vi "PC Send Event.vi"(0 "PC Send Command":T1, 2 "Mode":T2, 7 "Flattened Data":string, 11 "Error In":errorcluster) -> (4 "PC Send Event":refnum<user-event>, 15 "Error Out":errorcluster)   [LabVIEW 2019]
uses:
  Event Mode.ctl
  PCsend RTrecv CMD.ctl
  PCsend RTrecv Cluster.ctl
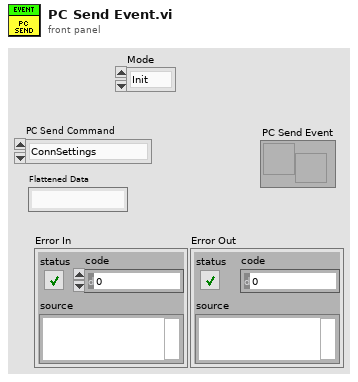
[diagram p1: front panel]
types:
  T1 = typedef "PCsend RTrecv CMD.ctl" = enum16{"ConnSettings", "Connect", "Stop", "Digital Outputs", "Analog Outputs", "Sweep Parameters", "Start Sweep", "Cal2RT", "Save Cal", "Load Cal"}
  T2 = typedef "Event Mode.ctl" = enum16{"Init", "Get", "Set", "Destroy"}
  T3 = typedef "PCsend RTrecv Cluster.ctl" = cluster{"PCsend/RTrecv CMD":T1, "Flattened Data":string}
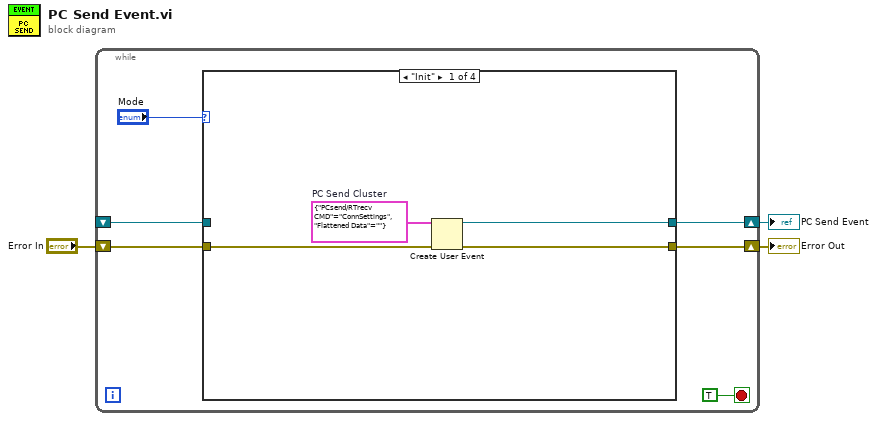
[diagram p0: block diagram]
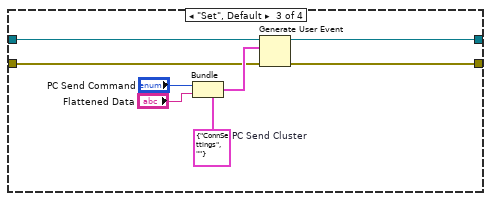
[diagram p3: hidden frame]
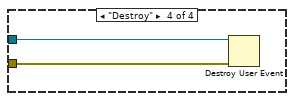
[diagram p4: hidden frame]
diagram:
  n1 = while {
    shift-right: [w7] -> w1
    shift-left: _ -> [w4]
    shift-right: [w6] -> w2
    shift-left: "Error In" -> [w5]
    stop <- TRUE stop-if-true
    n2 = case shown="\"Init\"" "Mode" {
      tunnel: [w12 w15 w16 _] -> w7
      tunnel: [w11 w14 w17 _] -> w6
      tunnel: w5 -> [w10 w14 w18 w24]
      tunnel: w4 -> [_ w15 w19 w25]
      frame "Init" {
        w13 = T3 {"PCsend/RTrecv CMD"=enum."ConnSettings", "Flattened Data"=""}  # PC Send Cluster
        n3 = Create User Event(user event datatype=w13, error in=w10) -> (user event=w12:refnum<user-event>, error out=w11:errorcluster)
      }
      frame "Get" {
      }
      frame "Set", Default {
        w20 = T3 {"PCsend/RTrecv CMD"=enum."ConnSettings", "Flattened Data"=""}  # PC Send Cluster
        n4 = Bundle(cluster=w20, "PCsend/RTrecv CMD"="PC Send Command", "Flattened Data"="Flattened Data") -> (w22:T3)
        n5 = Generate User Event(user event=w19, event data cluster=w22, error in=w18) -> (user event out=w16:refnum<user-event>, error out=w17:errorcluster)  [unwired: 1 in]
      }
      frame "Destroy" {
        n6 = Destroy User Event(user event=w25, error in=w24) -> ()  [unwired: 1 out]
      }
    }
  }
  "Error Out" <- w2
  "PC Send Event" <- w1
